vi "CLD 2  Elapsed Time Express Caller Solution.vi"() -> ()   [LabVIEW 2019]
doc: "CLD 2 Exercise \n\nThis VI is a wrapper used to call the FGV solution. The Express VI FGV can't be called directly because once the Express VI goes out of memory it can't track time. \n\nUsing the \"Get Time/Date\" or \"Tick Count\" primitives do not have this consideration."
uses:
  CLD 2 Time Mode.ctl
panel:
  out "Time Has Elapsed":bool
  out "Elapsed Time (s)":dbl format="%#.2g"
  out "error out":errorcluster
  in  "Time Target (s)":dbl=4.0
  in  "Auto Reset (F)":bool=TRUE
  in  "error in":errorcluster
  in  "Timer Mode":T1
  in  "stop":bool
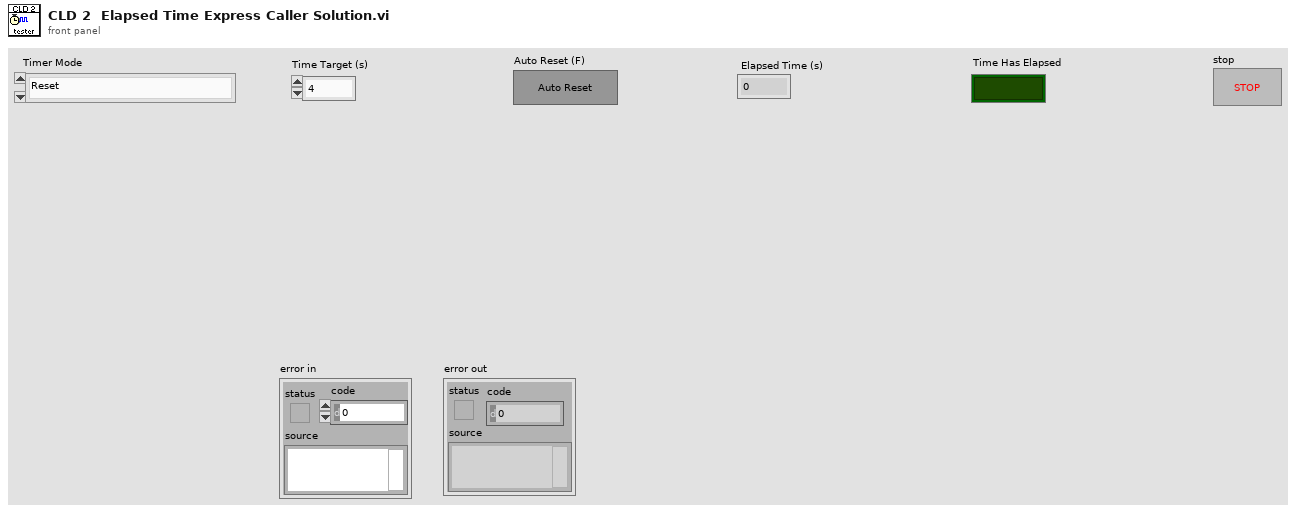
[diagram p1: front panel]
types:
  T1 = typedef "CLD 2 Time Mode.ctl" = enum16{"Reset", "Read Status", "Set Auto Reset"}
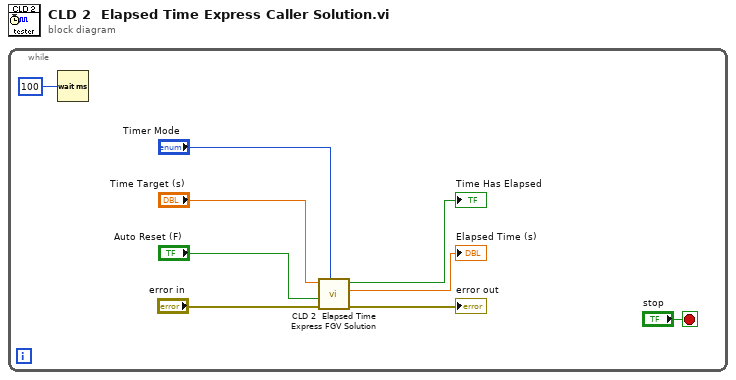
[diagram p0: block diagram]
diagram:
  n1 = while {
    stop <- "stop" stop-if-true
    n2 = Wait (ms)(milliseconds to wait=u32 100) -> ()  [unwired: 1 out]
    n3 = call "CLD 2  Elapsed Time Express FGV Solution.vi"("Timer  Mode"="Timer Mode", "error in (no error)"="error in", "Auto Reset (F)"="Auto Reset (F)", "Time Target (s)"="Time Target (s)") -> ("error out"=→"error out":errorcluster, "Elapsed Time (s)"=→"Elapsed Time (s)":dbl, "Time Has Elapsed"=→"Time Has Elapsed":bool)  [unwired: 5 in]
  }
